vi "getClosestIntersectionFromAttacker.vi"(9 "P2":dbl[](array[numeric]), 10 "P1":dbl[](array[numeric]), 11 "IA State Input":T1={"our_robots"=[], "enemy_robots"=[], "balls"=[], "geometry"={"line_width"=0, "field_length"=0, "field_width"=0, "boundary_width"=0, "referee_width"=0, "goal_width"=0, "goal_depth"=0, "goal_wall_width"=0, "center_circle_radius"=0, "defense_radius"=0, "defense_stretch"=0, "free_kick_from_defense_dist"=0, "penalty_spot_from_field_line_dist"=0, "penalty_line_from_spot_dist"=0}, "IA Judge"={"stage"="", "command"="", "our_goalie_id"=0.0, "enemy_goalie_id"=0.0, "command enum"=enum."Halt", "Time"=enum."Azul"}, "Received Timestamp"=timestamp(0 s since 1904-01-01), "Events"={"Touch"=FALSE, "Ball out"=FALSE, "id touch"=0.0, "Ball out of \nVision"=FALSE, "Ball inside \nGoalie area"=FALSE, "Robot not responding"=FALSE, "Robots responding status"=[1.0, 1.0, 1.0, 1.0, 1.0, 1.0], "Enemy Ball \nPossession"=FALSE, "Pass State"=FALSE, "id end of pass"=0.0, "Kick"=FALSE, "Id ini Possession"=0.0, "Ball Possesion"=FALSE, "Id Possesion"=0.0, "Direct Kick"=FALSE, "2nd Strk Ativo"=FALSE}}) -> (1 "distance enemy-attacker":dbl, 2 "collision ?":bool, 3 "point of collision":sgl[](array[numeric]))   [LabVIEW 2018]
uses:
  Core/AI Input.ctl
  Core/AI Robot.ctl
  Intel/Functions Enum.ctl
  Intel/AttackerStates.ctl
  Path Planning/RRT/PathDests.ctl
  Path Planning/RRT/PathDest.ctl
  Core/AI Ball.ctl
  Core/Field Size.ctl
  Core/AI Judge.ctl
  Intel/Command Enum.ctl
  Util/Events/Events.ctl
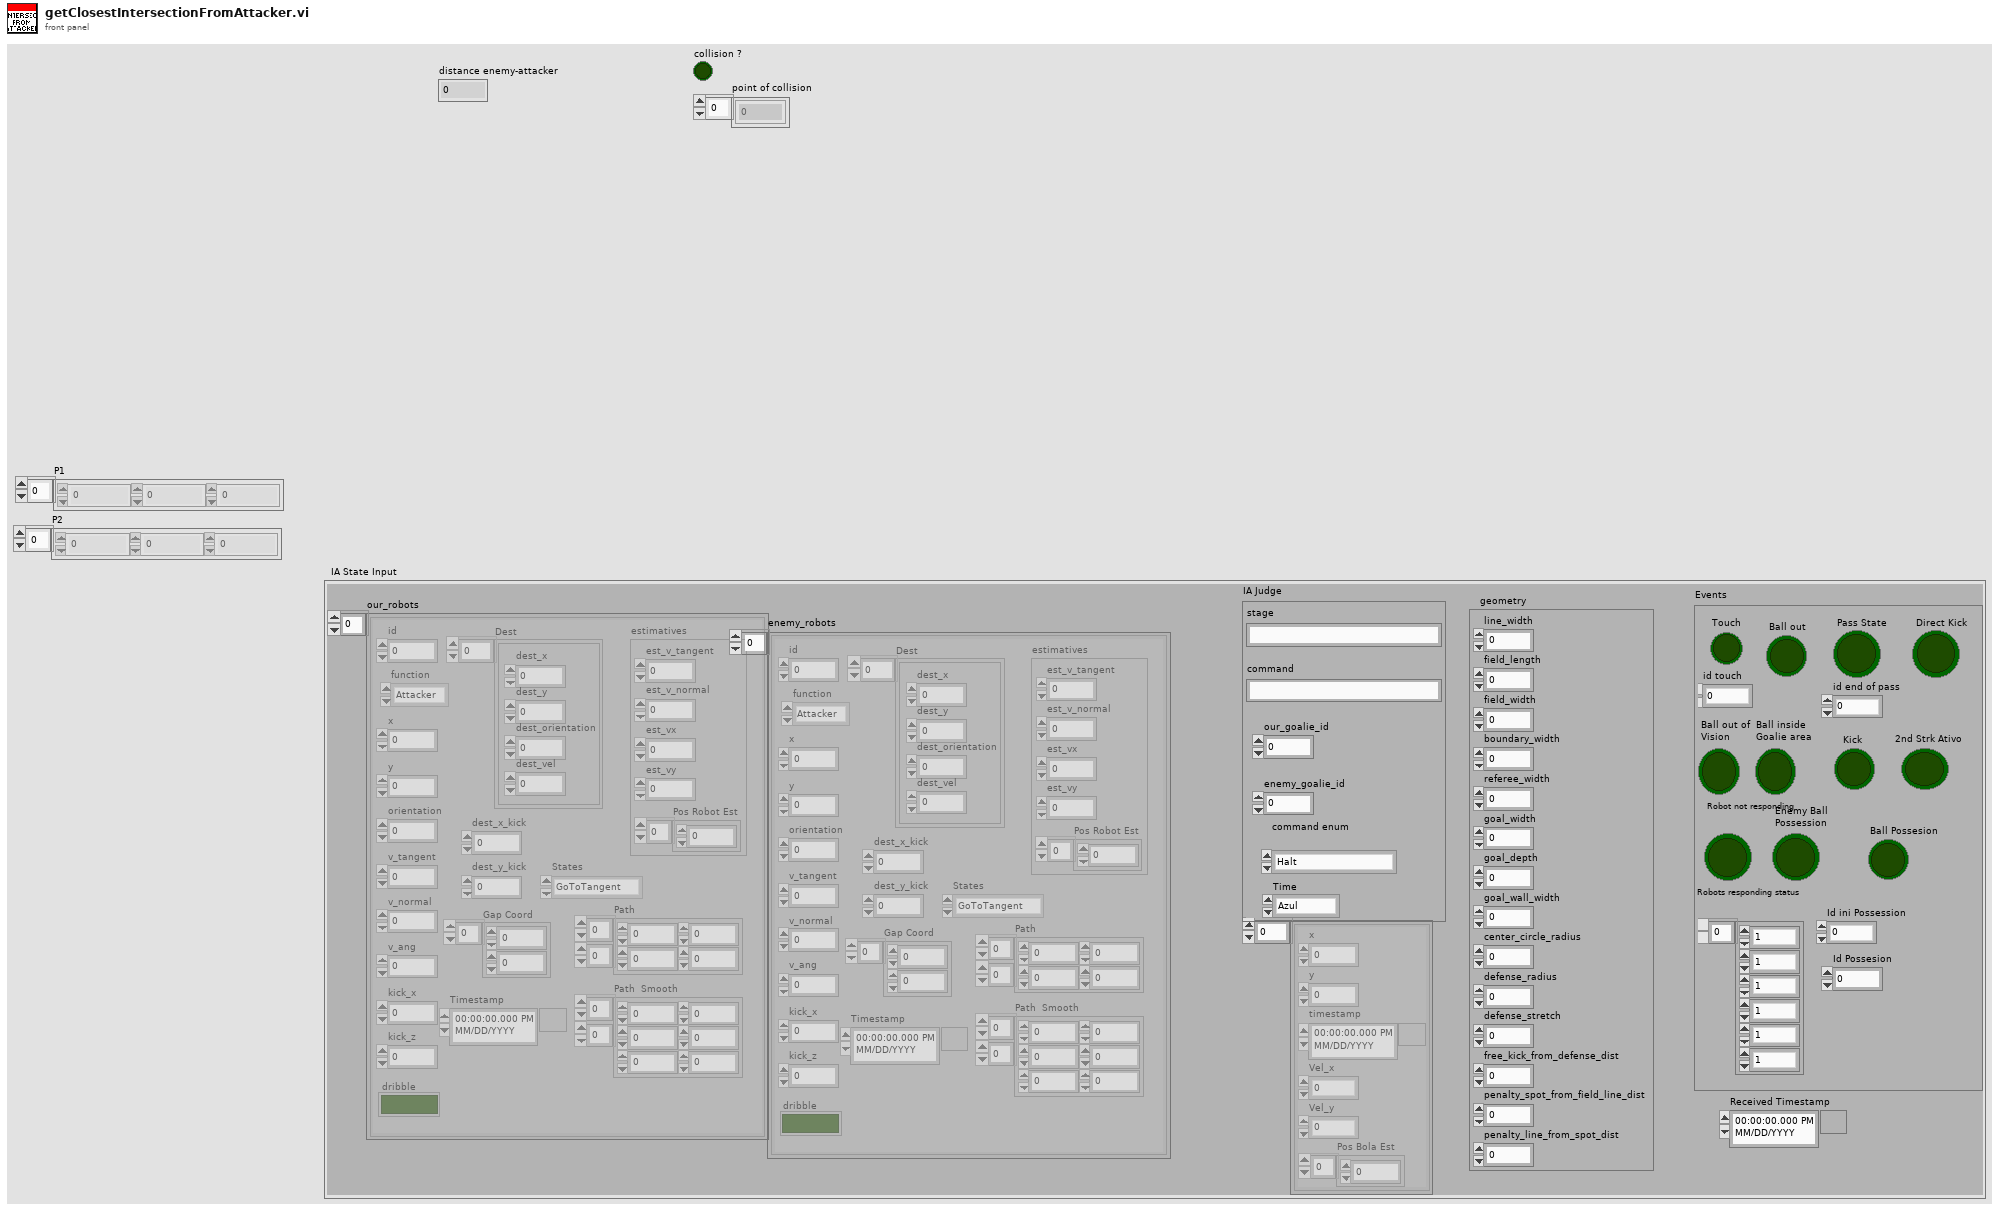
[diagram p1: front panel]
types:
  T1 = typedef "AI Input.ctl" = cluster{"our_robots":T2[], "enemy_robots":T2[], "balls":T7[], "geometry":T8, "IA Judge":T9, "Received Timestamp":timestamp, "Events":T11}
  T2 = typedef "AI Robot.ctl" = cluster{"id":u32, "function":T3, "x":dbl, "y":dbl, "orientation":dbl, "v_tangent":dbl, "v_normal":dbl, "v_ang":dbl, "kick_x":dbl, "kick_z":dbl, "dribble":bool, "Timestamp":timestamp, "estimatives":cluster{"est_v_tangent":dbl, "est_v_normal":dbl, "est_vx":dbl, "est_vy":dbl, "Pos Robot Est":dbl[]}, "dest_x_kick":dbl, "dest_y_kick":dbl, "Gap Coord":dbl[], "States":T4, "Path ":dbl[][], "Path  Smooth":dbl[][], "Dest":T5}
  T3 = typedef "Functions Enum.ctl" = enum16{"2nd Striker", "Attacker", "Goalie", "Defender", "Striker", "Goto 0", "Dummy", "Kicker", "ZigZag 0", "ZigZag 1", "ZigZag 2", "ZigZag 3", "ZigZag 4", "ZigZag 5", "ZigZag 6", "ZigZag 7", "ZigZag 8", ""}
  T4 = typedef "AttackerStates.ctl" = enum16{"Pass", "GoToTangent", "BallGetting", "GoToKick", ""}
  T5 = typedef "PathDests.ctl" = T6[]
  T6 = typedef "PathDest.ctl" = cluster{"dest_x":dbl, "dest_y":dbl, "dest_orientation":dbl, "dest_vel":dbl}
  T7 = typedef "AI Ball.ctl" = cluster{"x":dbl, "y":dbl, "timestamp":timestamp, "Vel_x":dbl, "Vel_y":dbl, "Pos Bola Est":dbl[]}
  T8 = typedef "Field Size.ctl" = cluster{"line_width":u32, "field_length":u32, "field_width":u32, "boundary_width":u32, "referee_width":u32, "goal_width":u32, "goal_depth":u32, "goal_wall_width":u32, "center_circle_radius":u32, "defense_radius":u32, "defense_stretch":u32, "free_kick_from_defense_dist":u32, "penalty_spot_from_field_line_dist":u32, "penalty_line_from_spot_dist":u32}
  T9 = typedef "AI Judge.ctl" = cluster{"stage":string, "command":string, "our_goalie_id":dbl, "enemy_goalie_id":dbl, "command enum":T10, "Time":enum16{"Azul", "Amarelo"}}
  T10 = typedef "Command Enum.ctl" = enum16{"Halt", "Stop", "Force Start", "PKA Normal Start", "Prepare Kickoff Ally", "PKE Normal Start", "Prepare Kickoff Enemy", "Prepare Penalty Ally", "PPA Normal Start", "Prepare Penalty Enemy", "PPE Normal Start", "Direct Free Enemy", "Direct Free Ally", "Indirect Free Enemy", "Indirect Free Ally", "Timeout Enemy", "Timeout Ally", "Goal Enemy", "Goal Ally", "Ball Placement Enemy", "Ball Placement Ally", "Normal Half Time", "Extra Time Break", "Extra Half Time", "None", "Post Game"}
  T11 = typedef "Events.ctl" = cluster{"Touch":bool, "Ball out":bool, "id touch":dbl, "Ball out of \nVision":bool, "Ball inside \nGoalie area":bool, "Robot not responding":bool, "Robots responding status":dbl[], "Enemy Ball \nPossession":bool, "Pass State":bool, "id end of pass":dbl, "Kick":bool, "Id ini Possession":dbl, "Ball Possesion":bool, "Id Possesion":dbl, "Direct Kick":bool, "2nd Strk Ativo":bool}
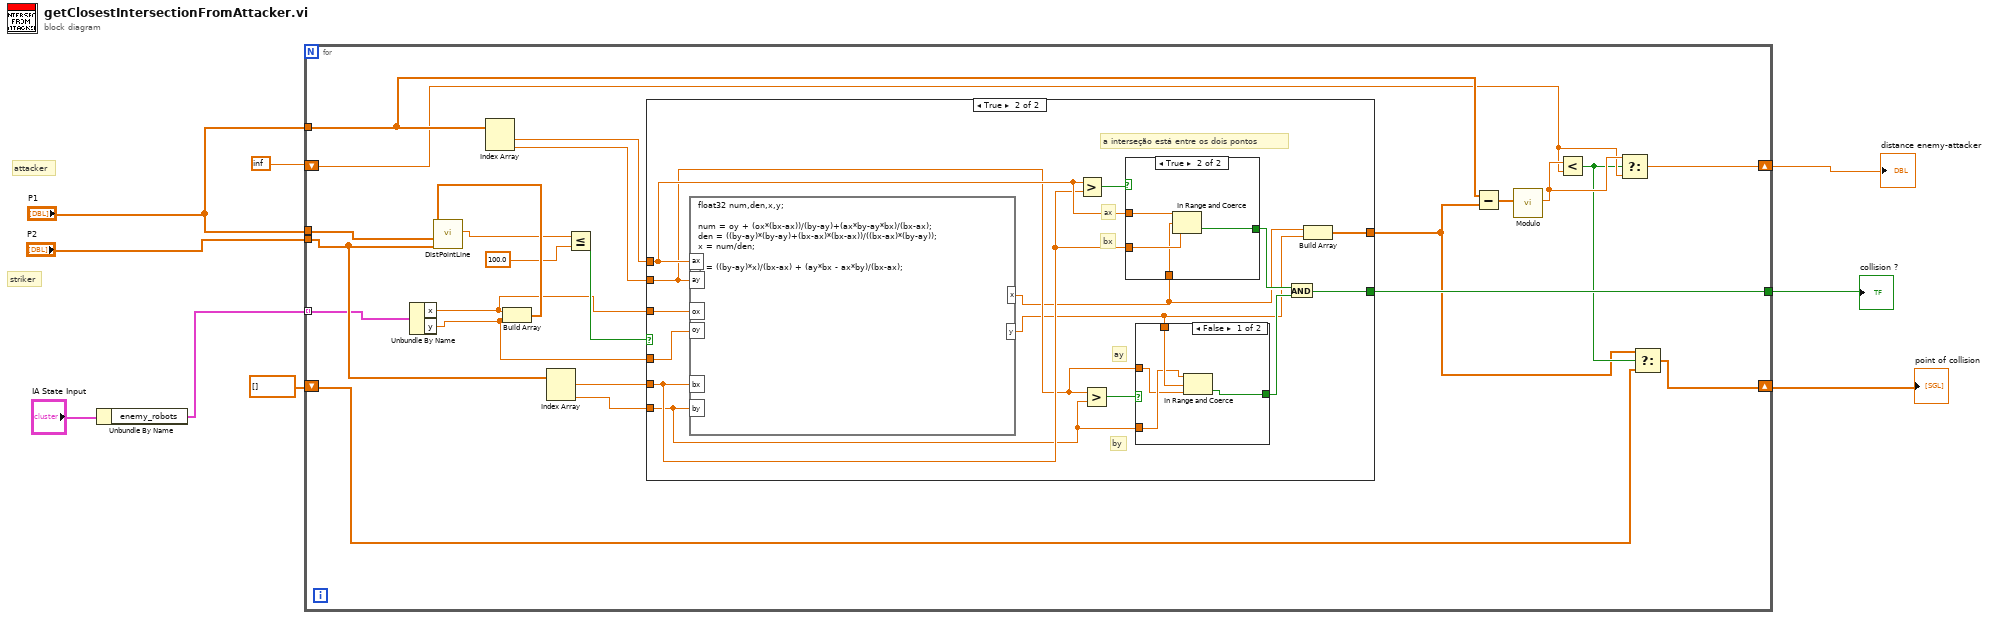
[diagram p0: block diagram]
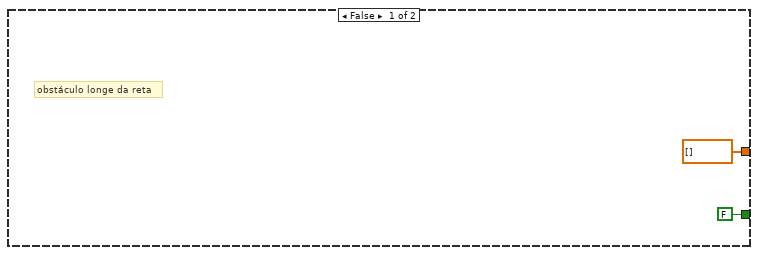
[diagram p2: hidden frame]
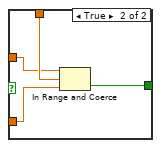
[diagram p3: hidden frame]
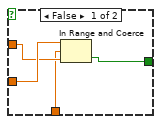
[diagram p4: hidden frame]
diagram:
  # "striker"
  # "attacker"
  n1 = Unbundle By Name("IA State Input") -> ("enemy_robots"=w4:T2[])
  n2 = for {
    tunnel: "P1" -> [w32]
    tunnel: "P2" -> [w25]
    tunnel: "P1" -> [w18]
    tunnel: [w22] -> w7
    tunnel: w4 -> [w21] mode=indexing
    shift-right: [w14] -> w1
    shift-left: inf -> [w15]
    shift-right: [w10] -> w6
    shift-left: sgl[] [] -> [w11]
    n3 = Unbundle By Name(w21) -> ("x"=w20:dbl, "y"=w19:dbl)
    n4 = Index Array(array=w18) -> (element #1=w27:dbl, element #2=w26:dbl)  [unwired: 2 in]
    n5 = Build Array(w20, w19) -> (w31:dbl[])
    n6 = call "DistPointLine.vi"("P2"=w25, "P1"=w32, "Q"=w31) -> ("distance"=w30:dbl)  [unwired: 8 in]
    n7 = Index Array(array=w25) -> (element #1=w24:dbl, element #2=w23:dbl)  [unwired: 2 in]
    n8 = Less Or Equal?(x=w30, y=100.0) -> (x <= y?=w28:bool)
    n9 = case shown="True" w28 {
      tunnel: w27 -> [_ w45]
      tunnel: w26 -> [_ w42]
      tunnel: w20 -> [_ w48]
      tunnel: w19 -> [_ w47]
      tunnel: w24 -> [_ w44]
      tunnel: w23 -> [_ w41]
      tunnel: [FALSE w38] -> w22
      tunnel: [sgl[] [] w35] -> w12
      frame False {
        # "obstáculo longe da reta"
      }
      frame True {
        # "a interseção está entre os dois pontos"
        # "by"
        # "ay"
        # "bx"
        # "ax"
        n10 = formula code="float32 num,den,x,y;\n\nnum = oy + (ox*(bx-ax))/(by-ay)+(ax*by-ay*bx)/(bx-ax);\nden = ((by-ay)*(by-ay)+(bx-ax)*(bx-ax))/((bx-ax)*(by-ay));\nx = num/den;\n\ny = ((by-ay)*x)/(bx-ax) + (ay*bx - ax*by)/(bx-ax);"("ax"=w45, "ay"=w42, "ox"=w48, "oy"=w47, "bx"=w44, "by"=w41) -> ("x"=w37:sgl, "y"=w36:sgl)
        n11 = Greater?(x=w45, y=w44) -> (0:w46:bool)
        n12 = Greater?(x=w42, y=w41) -> (0:w43:bool)
        n13 = case shown="True" w46 {
          tunnel: w45 -> [w59 w64]
          tunnel: w44 -> [w60 w63]
          tunnel: [w58 w62] -> w40
          tunnel: w37 -> [w57 w61]
          frame False {
            n14 = In Range and Coerce(upper limit=w60, x=w57, lower limit=w59) -> (In Range?=w58:bool)  [unwired: 1 out]
          }
          frame True {
            n15 = In Range and Coerce(upper limit=w64, x=w61, lower limit=w63) -> (In Range?=w62:bool)  [unwired: 1 out]
          }
        }
        n16 = case shown="False" w43 {
          tunnel: [w52 w56] -> w39
          tunnel: w42 -> [w49 w54]
          tunnel: w41 -> [w50 w53]
          tunnel: w36 -> [w51 w55]
          frame False {
            n17 = In Range and Coerce(upper limit=w50, x=w51, lower limit=w49) -> (In Range?=w52:bool)  [unwired: 1 out]
          }
          frame True {
            n18 = In Range and Coerce(upper limit=w54, x=w55, lower limit=w53) -> (In Range?=w56:bool)  [unwired: 1 out]
          }
        }
        n19 = And(x=w40, y=w39) -> (x .and. y?=w38:bool)
        n20 = Build Array(w37, w36) -> (w35:sgl[])
      }
    }
    n21 = Subtract(x=w18, y=w12) -> (x-y=w17:dbl[])
    n22 = call "Modulo.vi"("2D vector"=w17) -> ("Modulo"=w16:dbl)  [unwired: 10 in]
    n23 = Less?(x=w16, y=w15) -> (x < y?=w13:bool)
    n24 = Select(t=w16, s=w13, f=w15) -> (s? t:f=w14:dbl)
    n25 = Select(t=w12, s=w13, f=w11) -> (s? t:f=w10:sgl[])
  }
  "collision ?" <- w7
  "point of collision" <- w6
  "distance enemy-attacker" <- w1
